vi "RT Driver VI.vi"(7 "Operation":T1, 11 "Device Reference in":T2 format="%.0x") -> (0 "Error Code":i32)   [LabVIEW 2013, in "Trigger Timestamp Logging Engine.lvlib"]
uses:
  Trigger Timestamp Logging Engine.lvlib
  <vilib>/NI Veristand/Custom Device API/Custom Device Item Ref.ctl
  <vilib>/NI Veristand/Custom Device API/Hardware Interface Driver VI Operation.ctl
  <vilib>/xnet/xnet.llb/XNET Control Scope.ctl
  <vilib>/NI Veristand/Custom Device API/Get Item Property (Variant).vi
  <vilib>/NI Veristand/Custom Device API/Custom Device API.lvlib
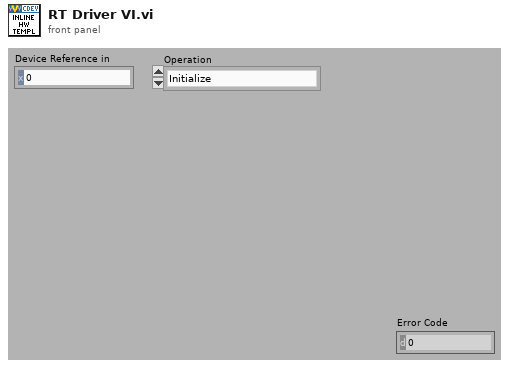
[diagram p1: front panel]
types:
  T1 = typedef "Custom Device API.lvlib/Hardware Interface Driver VI Operation.ctl" = enum16{"Initialize", "Start", "Read Data from HW", "Write Data to HW", "Close"}
  T2 = typedef "Custom Device API.lvlib/Custom Device Item Ref.ctl" = u64
  T3 = cluster{"Device Error":errorcluster, "Session1":refnum<k21>, "Session2":refnum<k21>}
  T4 = cluster{"Interface1":string, "Interface2":string, "Interface 1 DB":refnum<k21>, "Interface 2 DB":refnum<k21>}
  T5 = typedef "XNET Control Scope.ctl" = u32
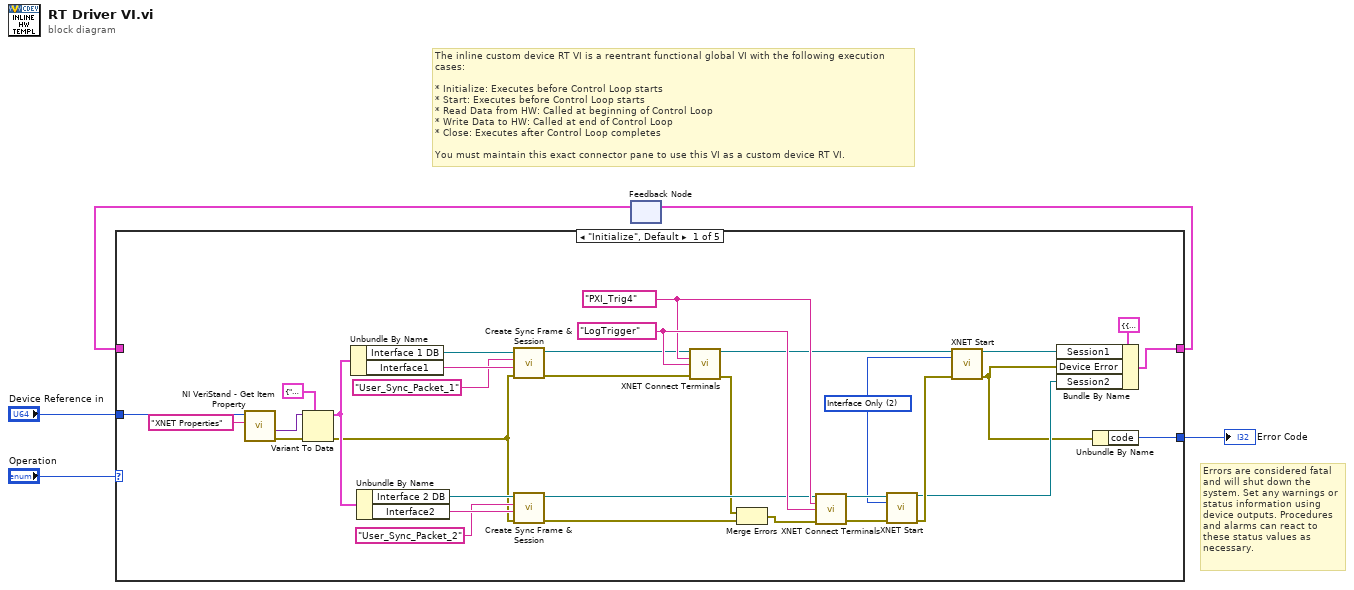
[diagram p0: block diagram]
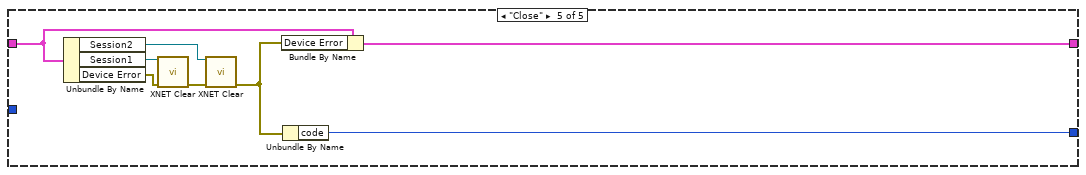
[diagram p5: hidden frame]
diagram:
  # "Errors are considered fatal and will shut down the system. Set any warnings or status information using device outputs. Procedures and alarms can react to these status values as necessary."
  # "The inline custom device RT VI is a reentrant functional global VI with the following execution cases:\n\n* Initialize: Executes before Control Loop starts\n* Start: Executes before Control Loop starts\n* Read Data from HW: Called at beginning of Control Loop\n* Write Data to HW: Called at end of Control Loop\n* Close: Executes after Control Loop completes\n\nYou must maintain this exact connector pane to use this VI as a custom device RT VI."
  n1 = feedback #1() -> (w3:T3)  [unwired: 1 out]
  n2 = case shown="\"Initialize\", Default" "Operation" {
    tunnel: [w36 w38 w39 w40 w41] -> w4
    tunnel: w3 -> [_ w38 w39 w40 w44]
    tunnel: "Device Reference in" -> [w37 _ _ _ _]
    tunnel: [w35 _ _ _ w42] -> w1
    frame "Initialize", Default {
      w23 = T5 2 items=["Normal", "Session Only", "Interface Only", "Session Only Blocking"] ("scope (normal)")
      w30 = tag "LogTrigger" ("NI-XNET Trigger Destination")
      w29 = tag "PXI_Trig4" ("NI-XNET Trigger source")
      n3 = call-poly <vilib>:"NI VeriStand - Get Item Property.vi"("Property Name"="XNET Properties", "Item Ref in"=w37) -> ("error out"=w32:errorcluster, "Value"=w33:variant)  [unwired: 6 in, 2 out]
      n4 = Variant To Data(error in=w32, type=T4 {"Interface1"="", "Interface2"="", "Interface 1 DB"="125kDB", "Interface 2 DB"="125kDB"}, Variant=w33) -> (data=w20:T4, error out=w10:errorcluster)
      n5 = Unbundle By Name(w20) -> ("Interface 1 DB"=w22:refnum<k21>, "Interface1"=w21:string)
      n6 = Unbundle By Name(w20) -> ("Interface 2 DB"=w13:refnum<k21>, "Interface2"=w12:string)
      n7 = call "Create Sync Frame & Session.vi"("error in (no error)"=w10, "Interface Name"=w21, "Sync Packet Name"="User_Sync_Packet_1" ("frame name"), "XNET Database Ref"=w22) -> ("error out"=w14:errorcluster, "Dummy XNET Session"=w28:refnum<k21>)  [unwired: 6 in]
      n8 = call "Create Sync Frame & Session.vi"("error in (no error)"=w10, "Interface Name"=w12, "Sync Packet Name"="User_Sync_Packet_2" ("frame name"), "XNET Database Ref"=w13) -> ("error out"=w6:errorcluster, "Dummy XNET Session"=w9:refnum<k21>)  [unwired: 6 in]
      n9 = call <vilib>:"XNET Connect Terminals.vi"("session in"=w28, "source terminal"=w29, "destination terminal"=w30, "error in (no error)"=w14) -> ("session out"=w25:refnum<k21>, "error out"=w7:errorcluster)  [unwired: 10 out]
      n10 = Merge Errors(w7, w6) -> (w8:errorcluster)
      n11 = call <vilib>:"XNET Connect Terminals.vi"("session in"=w9, "source terminal"=w29, "destination terminal"=w30, "error in (no error)"=w8) -> ("session out"=w26:refnum<k21>, "error out"=w27:errorcluster)  [unwired: 10 out]
      n12 = call <vilib>:"XNET Start.vi"("session in"=w26, "scope (normal)"=w23, "error in (no error)"=w27) -> ("session out"=w17:refnum<k21>, "error out"=w24:errorcluster)  [unwired: 11 out]
      n13 = call <vilib>:"XNET Start.vi"("session in"=w25, "scope (normal)"=w23, "error in (no error)"=w24) -> ("session out"=w18:refnum<k21>, "error out"=w16:errorcluster)  [unwired: 11 out]
      n14 = Bundle By Name(cluster=T3 {"Device Error"={"status"=FALSE, "code"=0, "source"=""}, "Session1"="", "Session2"=""}, "Session1"=w18, "Device Error"=w16, "Session2"=w17) -> (w36:T3)
      n15 = Unbundle By Name(w16) -> ("code"=w35:i32)
    }
    frame "Start" {
      # "Do Nothing"
    }
    frame "Read Data from HW" {
      # "Do Nothing"
    }
    frame "Write Data to HW" {
      # "Do Nothing"
    }
    frame "Close" {
      n16 = Unbundle By Name(w44) -> ("Session2"=w45:refnum<k21>, "Session1"=w48:refnum<k21>, "Device Error"=w47:errorcluster)
      n17 = call <vilib>:"XNET Clear.vi"("session in"=w48, "error in (no error)"=w47) -> ("error out"=w46:errorcluster)  [unwired: 13 out]
      n18 = call <vilib>:"XNET Clear.vi"("session in"=w45, "error in (no error)"=w46) -> ("error out"=w43:errorcluster)  [unwired: 13 out]
      n19 = Bundle By Name(cluster=w44, "Device Error"=w43) -> (w41:T3)
      n20 = Unbundle By Name(w43) -> ("code"=w42:i32)
    }
  }
  "Error Code" <- w1
  n21 = feedback-in #1(w4) -> ()
